vi "DHE_GetPixWriteTimeAlgors.vi"() -> (7 "writetimealgors":string[](array[string]))   [LabVIEW 2016]
uses:
  private/vis/DHE_VarAction.ctl
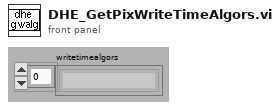
[diagram p1: front panel]
types:
  T1 = typedef "DHE_VarAction.ctl" = enum16{"read", "write"}
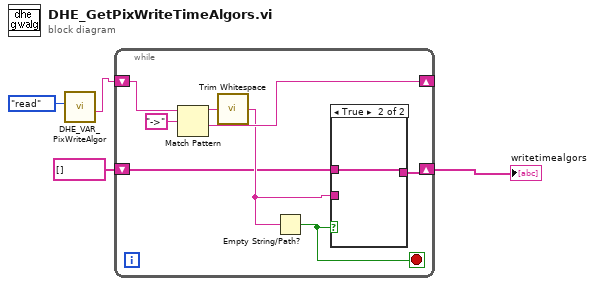
[diagram p0: block diagram]
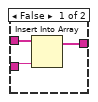
[diagram p2: hidden frame]
diagram:
  n1 = call "DHE_VAR_PixWriteAlgor.vi"("action"=DHE_VarAction."read") -> ("PixReadAlgors"=w1:string)  [unwired: 1 in, 9 out]
  n2 = while {
    shift-right: [w11] -> _
    shift-left: w1 -> [w5]
    shift-right: [w7] -> w2
    shift-left: string[] [] -> [w6]
    stop <- w9 stop-if-true
    n3 = Match Pattern(string=w5, regular expression="->") -> (before substring=w10:string, after substring=w11:string)  [unwired: 3 out]
    n4 = call <vilib>:"Trim Whitespace.vi"("string"=w10) -> ("trimmed string"=w8:string)  [unwired: 1 in]
    n5 = Empty String/Path?(string/path=w8) -> (empty?=w9:bool)
    n6 = case shown="True" w9 {
      tunnel: w8 -> [w15 _]
      tunnel: [w14 w16] -> w7
      tunnel: w6 -> [w13 w16]
      frame False {
        n7 = Insert Into Array(array=w13, new element=w15) -> (w14:string[])  [unwired: 1 in]
      }
      frame True {
      }
    }
  }
  "writetimealgors" <- w2
